vi "test SGL type.vi"() -> ()   [LabVIEW 2017]
uses:
  <resource>/objmgr/ni.var.rc
  Scan Engine Custom Device.lvlib
panel:
  out "element":i16
  out "32bit integer":i32 format="%.0x"
  out "UDV Data Type":string
  out "Data Type":variant
  out "Writable":bool
  out "Name":string
  out "shared variable refnum in":refnum<k21>
  out "error out":errorcluster
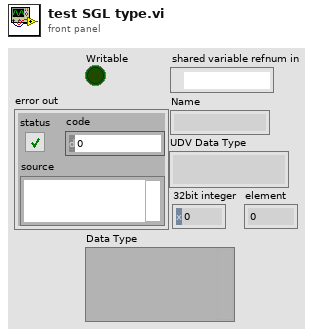
[diagram p1: front panel]
types:
  T1 = typedef "Scan Engine Custom Device.lvlib/ECAT Channel Data Type.ctl" = enum16{"Boolean", "Fixed Point", "Int8", "Int16", "Int32", "Int64", "U32 Bit Field", "UInt8", "UInt16", "UInt32", "UInt64", "Other", "DBL", "SGL"}
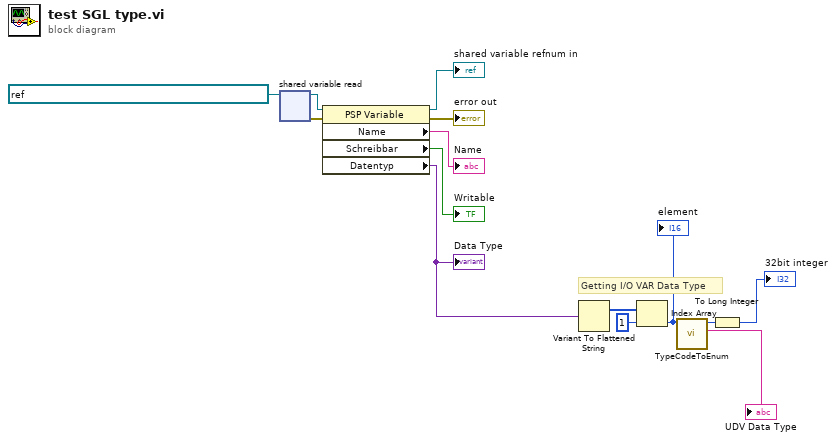
[diagram p0: block diagram]
diagram:
  # "Getting I/O VAR Data Type"
  n1 = shared-variable-read(refnum<k21> "ni.var.psp://my computer/LibTest/Variable1" ("shared variable refnum in")) -> (w13:refnum<k21>, w12:errorcluster)  [unwired: 1 in, 1 out]
  n2 = property class="PSP Variable"(reference=w13, error in=w12) -> (reference out=→"shared variable refnum in":refnum<k21>, error out=→"error out":errorcluster, "Name"=→"Name":string, "Schreibbar"=→"Writable":bool, "Datentyp"=w3:variant)
  "Data Type" <- w3
  n3 = Variant To Flattened String(Variant=w3) -> (1:w4:i16[])  [unwired: 1 out]
  n4 = Index Array(array=w4, index=1) -> (element=w6:i16)
  "element" <- w6
  n5 = call "TypeCodeToEnum.vi"("Type Code (numbers in hexadecimal)"=w6) -> (2:"UDV Data Type"=→"UDV Data Type":string, 3:"UDV Data Type"=w7:T1)  [unwired: 9 in]
  n6 = To Long Integer(number=w7) -> (32bit integer=→"32bit integer":i32)
